vi "Sweep Step Ring to MHz.vi"(10 "Frequency Increment Ring":u32(ring) items=["0.2", "0.4", "1.0", "2.0", "4.0"]) -> (2 "Frequency Increment MHz":dbl)   [LabVIEW 2011]
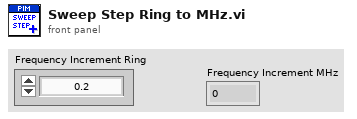
[diagram p1: front panel]
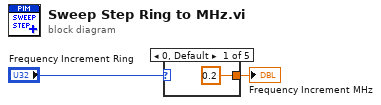
[diagram p0: block diagram]
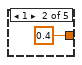
[diagram p2: hidden frame]
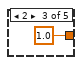
[diagram p3: hidden frame]
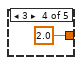
[diagram p4: hidden frame]
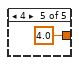
[diagram p5: hidden frame]
diagram:
  n1 = case shown="0, Default" "Frequency Increment Ring" {
    tunnel: [0.2 0.4 1.0 2.0 4.0] -> w1
    frame 0, Default {
    }
    frame 1 {
    }
    frame 2 {
    }
    frame 3 {
    }
    frame 4 {
    }
  }
  "Frequency Increment MHz" <- w1
